vi "Read Gas List.vi"(7 "Unit ID (A)":string="A", 8 "error in":errorcluster, 11 "VISA Session In":refnum<visa-resource-name>="Alicat") -> (0 "error out":errorcluster, 1 "Gas Selection: Strings and Values":cluster{"Gas Name":string, "Gas number":u16}[](array[cluster]), 2 "Gas Names":string[](array[string]), 3 "VISA Session Out":refnum<visa-resource-name>)   [LabVIEW 2016]
doc: "Outputs an array of gas names and numbers (paired for use with an arbitrary gas list, including custom mixes). The output \"Gas Selection: Strings and Values\" can be used with the \"Strings and Values\" property of a write property node linked to a ring control on the front panel to provide a ring control populated with the gas names."
uses:
  <vilib>/Instr/_visa.llb/VISA Flush IO Buffer Mask.ctl
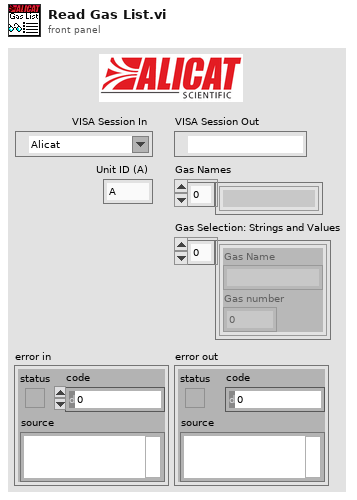
[diagram p1: front panel]
types:
  T1 = typedef "VISA Flush IO Buffer Mask.ctl" = u16
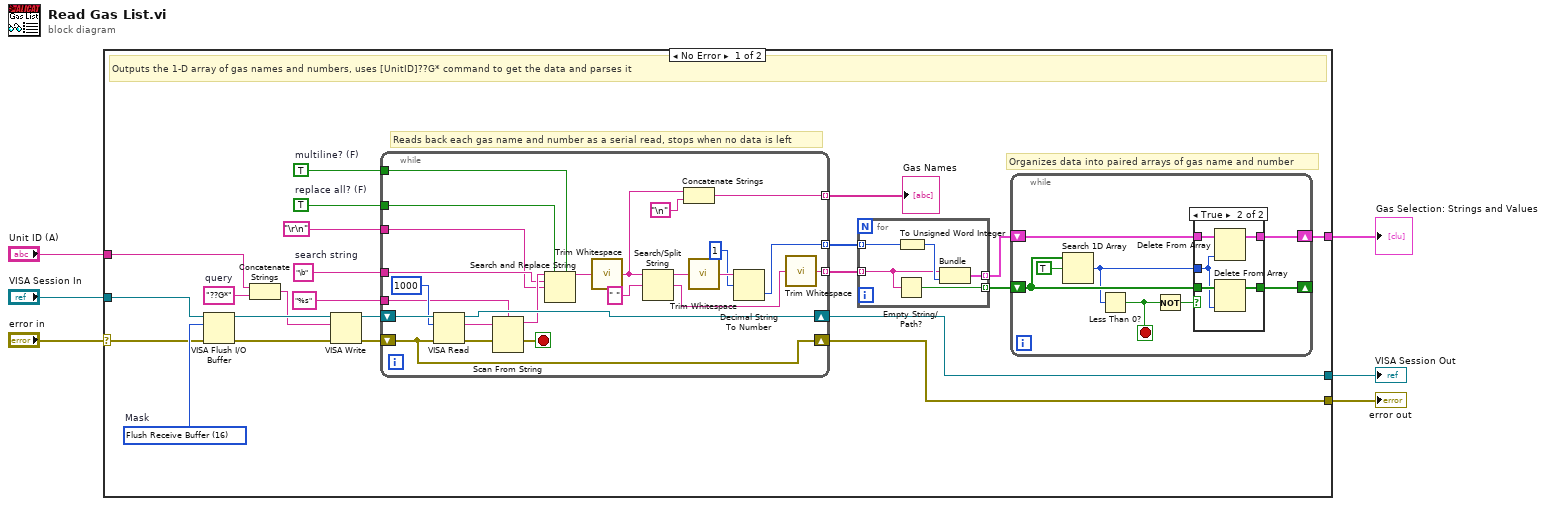
[diagram p0: block diagram]
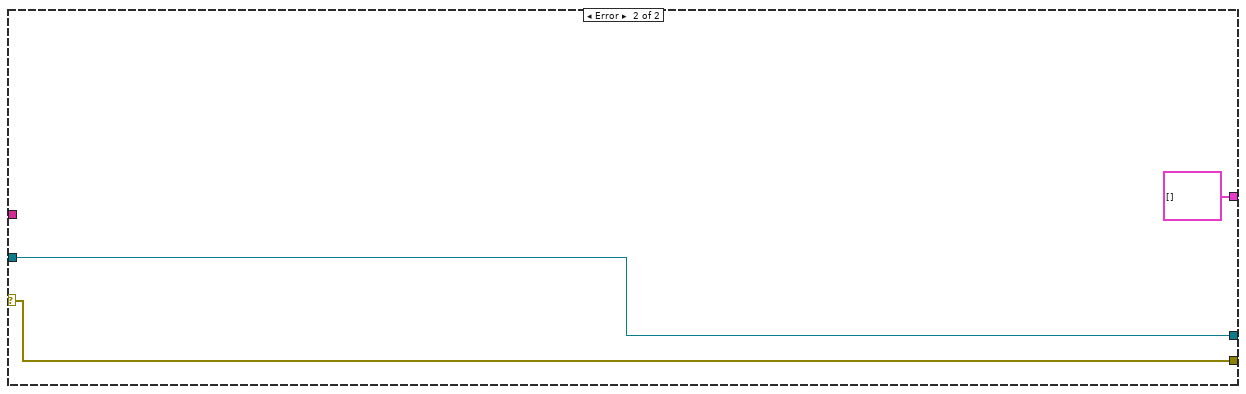
[diagram p3: hidden frame]
diagram:
  n1 = case shown="No Error" "error in" {
    selector: "error in" -> [w7 w74]
    tunnel: "VISA Session In" -> [w28 w76]
    tunnel: "Unit ID (A)" -> [w21 _]
    tunnel: [w15 w74] -> w4
    tunnel: [w14 w76] -> w3
    tunnel: [w9 cluster{"trimmed string":string, u16}[] []] -> w2
    frame No Error {
      w20 = TRUE  # multiline? (F)
      w19 = TRUE  # replace all? (F)
      w18 = "\b"  # search string
      w23 = "??G*"  # query
      w26 = T1 16 items=["Flush Receive Buffer"=16, "Write Transmit Buffer to Device"=32, "Flush Receive Buffer (No I/O)"=64, "Flush Transmit Buffer"=128]  # Mask
      # "Organizes data into paired arrays of gas name and number"
      # "Reads back each gas name and number as a serial read, stops when no data is left"
      # "Outputs the 1-D array of gas names and numbers, uses [UnitID]??G* command to get the data and parses it"
      n2 = VISA Flush I/O Buffer(VISA resource name=w28, mask (16)=w26, error in (no error)=w7) -> (VISA resource name out=w27:refnum<visa-resource-name>, error out=w24:errorcluster)
      n3 = Concatenate Strings(w21, w23) -> (w22:string)
      n4 = VISA Write(VISA resource name=w27, write buffer=w22, error in (no error)=w24) -> (VISA resource name out=w25:refnum<visa-resource-name>, error out=w29:errorcluster)  [unwired: 1 out]
      n5 = while {
        tunnel: [w61] -> w16 mode=indexing
        shift-right: [w50] -> w15
        shift-left: w29 -> [w50]
        shift-right: [w71] -> w14
        shift-left: w25 -> [w73]
        tunnel: w20 -> [w66]
        tunnel: w19 -> [w65]
        tunnel: w18 -> [w64]
        tunnel: "%s" ("format string") -> [w63]
        tunnel: [w55] -> w10 mode=indexing
        tunnel: [w58] -> w11 mode=indexing
        tunnel: "\r\n" -> [w51]
        stop <- w67 stop-if-true
        n6 = VISA Read(VISA resource name=w73, byte count=u32 1000, error in (no error)=w50) -> (VISA resource name out=w71:refnum<visa-resource-name>, read buffer=w70:string, error out=w72:errorcluster)  [unwired: 1 out]
        n7 = Scan From String(format string=w63, input string=w70, error in=w72) -> (remaining string=w68:string, error out=w67:errorcluster)  [unwired: 3 in, 1 out]
        n8 = Search and Replace String(replace all?=w65, multiline?=w66, input string=w68, search string=w64, replace string=w51) -> (result string=w62:string)  [unwired: 3 in, 3 out]
        n9 = call <vilib>:"Trim Whitespace.vi"("string"=w62) -> ("trimmed string"=w54:string)  [unwired: 1 in]
        n10 = Search/Split String(string=w54, search string/char (-)=" ") -> (substring before match=w53:string, match + rest of string=w59:string)  [unwired: 1 in, 1 out]
        n11 = Concatenate Strings(w54, "\n") -> (w61:string)
        n12 = call <vilib>:"Trim Whitespace.vi"("string"=w53) -> ("trimmed string"=w57:string)  [unwired: 1 in]
        n13 = Decimal String To Number(string=w57, offset=1) -> (number=w55:i32)  [unwired: 1 in, 1 out]
        n14 = call <vilib>:"Trim Whitespace.vi"("string"=w59) -> ("trimmed string"=w58:string)  [unwired: 1 in]
      }
      "Gas Names" <- w16
      n15 = for {
        tunnel: w10 -> [w48] mode=indexing
        tunnel: w11 -> [w46] mode=indexing
        tunnel: [w49] -> w12 mode=indexing
        tunnel: [w45] -> w13 mode=indexing
        n16 = Empty String/Path?(string/path=w46) -> (empty?=w45:bool)
        n17 = To Unsigned Word Integer(number=w48) -> (unsigned 16bit integer=w47:u16)
        n18 = Bundle("trimmed string"=w46, w47) -> (w49:cluster{"trimmed string":string, u16})  [unwired: 1 in]
      }
      n19 = while {
        shift-right: [w33] -> w9
        shift-left: w12 -> [w36]
        shift-right: [w32] -> _
        shift-left: w13 -> [w31]
        stop <- w35 stop-if-true
        n20 = Search 1D Array(1D array=w31, element=TRUE) -> (index of element=w30:i32)  [unwired: 1 in]
        n21 = Less Than 0?(x=w30) -> (x < 0?=w35:bool)
        n22 = Not(x=w35) -> (.not. x?=w34:bool)
        n23 = case shown="True" w34 {
          tunnel: w36 -> [w39 w44]
          tunnel: [w39 w43] -> w33
          tunnel: [w38 w42] -> w32
          tunnel: w31 -> [w38 w41]
          tunnel: w30 -> [_ w40]
          frame False {
          }
          frame True {
            n24 = Delete From Array(array=w44, index=w40) -> (array with subset deleted=w43:cluster{"trimmed string":string, u16}[])  [unwired: 1 in, 1 out]
            n25 = Delete From Array(array=w41, index=w40) -> (array with subset deleted=w42:bool[])  [unwired: 1 in, 1 out]
          }
        }
      }
    }
    frame Error {
    }
  }
  "error out" <- w4
  "VISA Session Out" <- w3
  "Gas Selection: Strings and Values" <- w2
